vi "Read Status.vi"(11 "Assertion Result In":refnum<class "Assertion Result.lvclass">) -> (2 "Status":T1, 3 "Assertion Result Out":refnum<class "Assertion Result.lvclass">)   [LabVIEW 2020, in "Assertion Result.lvclass"]
uses:
  Assertion Result.lvclass
  TypeDefs/Status.ctl
  Assertion Result.lvclass/Assertion Result.ctl
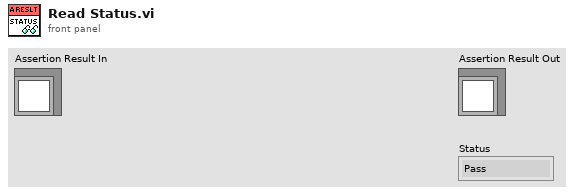
[diagram p1: front panel]
types:
  T1 = typedef "Assertion Result.lvclass/Status.ctl" = enum16{"Pass", "Fail", "Error", "Skipped", "Setup Error", "Broken", "Teardown Error"}
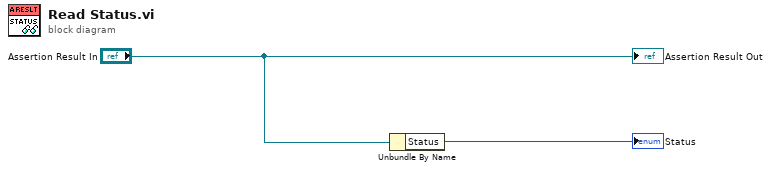
[diagram p0: block diagram]
diagram:
  n1 = Unbundle By Name("Assertion Result In") -> ("Status"=→"Status":T1)
  "Assertion Result Out" <- "Assertion Result In"
